vi "Make Stacks.vi"(10 "Stacks in":string[](array[string]), 11 "Labels":string[](array[string])) -> (3 "Stacks out":cluster{"Label":string, "Stack":string[]}[](array[cluster]))   [LabVIEW 2021]
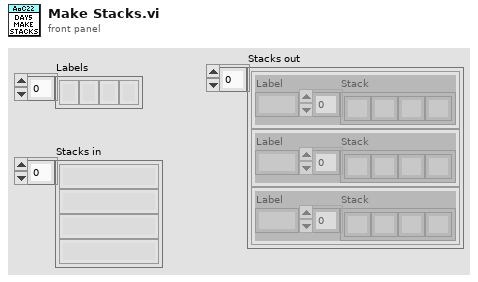
[diagram p1: front panel]
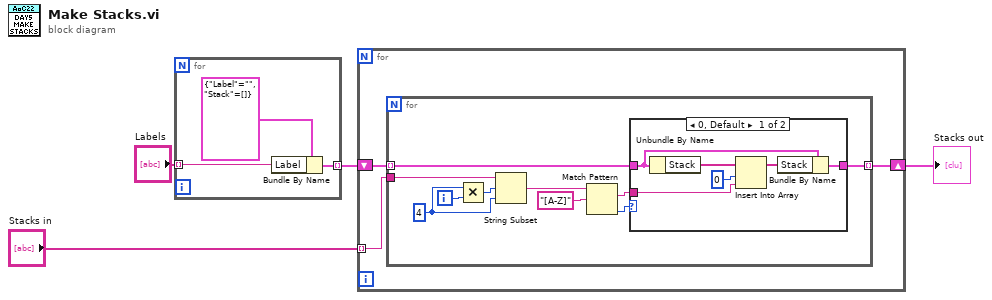
[diagram p0: block diagram]
diagram:
  n1 = for {
    tunnel: "Labels" -> [w7] mode=indexing
    tunnel: [w6] -> w3 mode=indexing
    n2 = Bundle By Name(cluster=cluster{"Label":string, "Stack":string[]} {"Label"="", "Stack"=[]}, "Label"=w7) -> (w6:cluster{"Label":string, "Stack":string[]})
  }
  n3 = for {
    tunnel: "Stacks in" -> [w10] mode=indexing
    shift-right: [w9] -> w4
    shift-left: w3 -> [w8]
    n4 = for {
      tunnel: w10 -> [w20]
      tunnel: [w13] -> w9 mode=indexing
      tunnel: w8 -> [w12] mode=indexing
      i -> [w18]
      w19 = 4 ("length (rest)")
      n5 = Multiply(x=w19, y=w18) -> (x*y=w17:i32)
      n6 = String Subset(string=w20, offset (0)=w17, length (rest)=w19) -> (substring=w16:string)
      n7 = Match Pattern(string=w16, regular expression="[A-Z]") -> (match substring=w11:string, offset past match=w14:i32)  [unwired: 1 in, 2 out]
      n8 = case shown="0, Default" w14 {
        tunnel: w12 -> [w26 w27]
        tunnel: [w25 w27] -> w13
        tunnel: w11 -> [w23 _]
        frame 0, Default {
          n9 = Unbundle By Name(w26) -> ("Stack"=w24:string[])
          n10 = Insert Into Array(array=w24, index=0, new element=w23) -> (w21:string[])
          n11 = Bundle By Name(cluster=w26, "Stack"=w21) -> (w25:cluster{"Label":string, "Stack":string[]})
        }
        frame -1 {
        }
      }
    }
  }
  "Stacks out" <- w4
